vi "LDA_Results_Row_info.vi"() -> (0 "Row Values":string[](array[string]), 1 "Row Headers":string[](array[string]))   [LabVIEW 2022 SP3]
uses:
  Globals/LDA_global.vi
  Globals/LDA_meas_global_1.vi
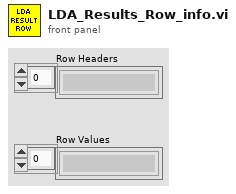
[diagram p1: front panel]
types:
  T1 = typedef "LDA_Channel.ctl" = cluster{"Wavelength (nm)":dbl, "Vel Comp":string, "Max Velocity":dbl, "Min Velocity":dbl, "Max Record length":u16, "Signal gain (dB)":i16, "High voltage":i16, "Optics Conversion Factor":dbl, "Min Record length":u16, "Multiply Velocity by -1":bool, "Signal to Noise Ratio":string, "Validation Ratio":string, "Probe":string, "Laser":string, "BSA":string, "Lense":string, "Beam Separation (mm)":dbl, "Focal Length (mm)":dbl, "COLOUR":u32, "BSA IP":string, "Velocity Range (m/s)":dbl, "Centre Velocity (m/s)":dbl, "Unshifted mW":dbl, "Shifted mW":dbl, "Bandwidth Hz":dbl, "Req Sampling Rate Hz":dbl, "Ch":i32, "CenterFreq Hz":dbl, "Laser IP":string, "Sync Delay (s)":dbl}
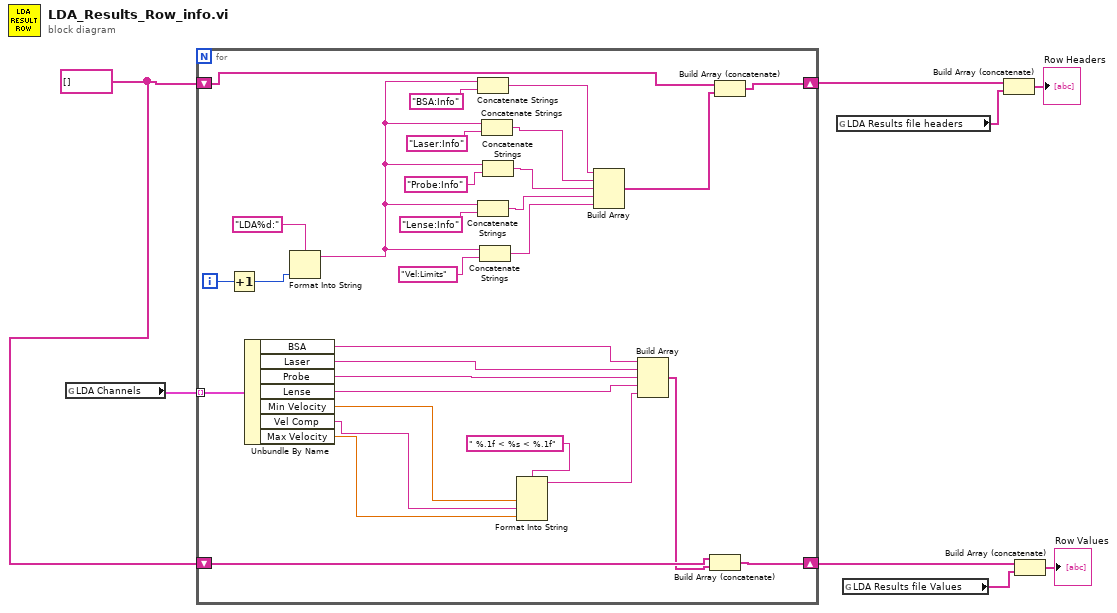
[diagram p0: block diagram]
diagram:
  w7 = string[] []
  n1 = global read "LDA_global.vi" "LDA Channels"() -> (w8:T1[])
  n2 = for {
    tunnel: w8 -> [w38] mode=indexing
    shift-right: [w13] -> w1
    shift-left: w7 -> [w12]
    shift-right: [w10] -> w6
    shift-left: w7 -> [w11]
    i -> [w28]
    n3 = Increment(x=w28) -> (x+1=w27:i32)
    n4 = Unbundle By Name(w38) -> ("BSA"=w33:string, "Laser"=w32:string, "Probe"=w31:string, "Lense"=w30:string, "Min Velocity"=w36:dbl, "Vel Comp"=w35:string, "Max Velocity"=w37:dbl)
    n5 = Format Into String(format string="LDA%d:", w27) -> (resulting string=w20:string)  [unwired: 2 in, 1 out]
    n6 = Concatenate Strings(w20, "BSA:Info" ("string")) -> (w19:string)
    n7 = Concatenate Strings(w20, "Lense:Info" ("string")) -> (w16:string)
    n8 = Concatenate Strings(w20, "Vel:Limits" ("string")) -> (w15:string)
    n9 = Concatenate Strings(w20, "Laser:Info" ("string")) -> (w18:string)
    n10 = Concatenate Strings(w20, "Probe:Info" ("string")) -> (w17:string)
    n11 = Format Into String(format string=" %.1f < %s < %.1f" ("Format String"), w36, w35, w37) -> (resulting string=w29:string)  [unwired: 2 in, 1 out]
    n12 = Build Array(w19, w18, w17, w16, w15) -> (w14:string[])
    n13 = Build Array(w33, w32, w31, w30, w29) -> (w9:string[])
    n14 = Build Array (concatenate)(w11, w9) -> (w10:string[])
    n15 = Build Array (concatenate)(w12, w14) -> (w13:string[])
  }
  n16 = global read "LDA_meas_global_1.vi" "LDA Results file headers"() -> (w2:string[])
  n17 = global read "LDA_meas_global_1.vi" "LDA Results file Values"() -> (w5:string[])
  n18 = Build Array (concatenate)(w1, w2) -> (→"Row Headers":string[])
  n19 = Build Array (concatenate)(w6, w5) -> (→"Row Values":string[])
